vi "write RT config file.vi"(9 "RT config":T18={"Message"={"Parameters"={"FPGA Ref"=refnum, "configID"=0, "activeChannels"=[]}, "Variables"={"RT Status"={"Comms loop"=FALSE, "scheduler loop"=FALSE, "data process loop"=FALSE, "FIFO loop"=FALSE, "Command Stream"=FALSE, "Error Stream"=FALSE, "FPGA FIFO"=FALSE, "Data Stream"=FALSE}, "watchdog"=timestamp(0 s since 1904-01-01), "limitsEnabled"=FALSE, "Interlocks"={"gearboxOil"=FALSE, "bearingOil"=FALSE, "gearboxAir"=FALSE}}}, "FIFO"={"Params"={"FPGA ref"=refnum, "Total Channels"=0}, "Variables"={"FIFO wait counter"=0, "FIFO read trigger"=0}}, "Comms data"={"Parameters"={"error writer name"="", "command reader name"="", "error buffer size"=0, "command buffer size"=0, "scanivalveIP"="", "scanivalvePeriod"=0}, "Variables"={"listen schedule"=0, "incident buffer"=[], "command stream"="", "error stream"="", "waiting for command stream connect"=FALSE, "waiting for error stream connect"=FALSE, "scanivalve connection"=refnum, "scanivalveScheduleID"=0, "activeScanivalvePorts"=[], "channelCount"=0}, "scanivalveConfig"={"listS"={"period"=0, "ADtrig"=FALSE, "ScanTrig"=FALSE, "page"=0, "qpkts"=0}, "listC"={"ZC"=FALSE, "unitScan"="", "CvtUnit"=0.0, "bin"=FALSE, "EU"=FALSE}, "listSG"={"Avg1"=0, "FPS1"=0, "SGEnable1"=FALSE}, "activeChannels"={"Chan1"={"101"=FALSE, "102"=FALSE, "103"=FALSE, "104"=FALSE, "109"=FALSE, "110"=FALSE, "111"=FALSE, "112"=FALSE, "201"=FALSE, "202"=FALSE, "203"=FALSE, "204"=FALSE, "209"=FALSE, "210"=FALSE, "211"=FALSE, "212"=FALSE, "301"=FALSE, "302"=FALSE, "303"=FALSE, "304"=FALSE, "309"=FALSE, "310"=FALSE, "311"=FALSE, "312"=FALSE, "401"=FALSE, "402"=FALSE, "403"=FALSE, "404"=FALSE, "409"=FALSE, "410"=FALSE, "411"=FALSE, "412"=FALSE}}}}, "Data processor"={"Parameters"={"FPGA Ref"=refnum, "data stream"={"data writer name"="error writer", "NS write buffer size"=16, "NS Buffer length"=0}, "FIFO Depth"=0, "Channel controls"={"FIFO channel count"=0, "active indices"=[], "active channels"=0, "channelScaling"=[], "scanivalveCount"=0, "channels"=[]}, "safetyChannels"={"oilP"=0, "airP"=0, "water"=0, "channelLimits"=[]}, "speedChannel"=0, "maxSpeedLimit"=0.0, "Torque"={"fixedOffset"=0.0, "filter"=FALSE, "fallingEdge"=FALSE, "swapEncoders"=FALSE}}, "Variables"={"Intermediary buffer"=[], "buffer position"=0, "write loop counter"=0, "NS write trigger"=0, "NS Connection status"=FALSE, "waiting for NS"=FALSE, "labAmbient"={"pressure"=0.0, "temperature"=0.0}, "scanivalvePorts"=[], "scanivalvePressures"=[], "data stream"="", "activeChannelLimitIndex"=[], "runningSpeedLimit"=0.0, "speedChannelIndex"=0, "Interlocks"={"gearboxOil"=FALSE, "bearingOil"=FALSE, "gearboxAir"=FALSE}, "interlockChannels"={"gearboxOil"=0, "bearingOil"=0, "air"=0}, "limitStates"=[]}}}, 11 "RT config file path":path) -> ()   [LabVIEW 2018]
uses:
  RT/Type Defs/Message loop data.ctl
  RT/Type Defs/FPGA reference.ctl
  RT/Type Defs/RT Status.ctl
  RT/Type Defs/Analogue loop data.ctl
  RT/Communications loop/comms data.ctl
  RT/Type Defs/generic incident.ctl
  ICL-LabVIEW_General/Scanivalve API project/full interface/polymorphic/scanivalveConfig.ctl
  ICL-LabVIEW_General/Scanivalve API project/full interface/listS.ctl
  ICL-LabVIEW_General/Scanivalve API project/full interface/listC.ctl
  ICL-LabVIEW_General/Scanivalve API project/full interface/listSG.ctl
  ICL-LabVIEW_General/Scanivalve API project/full interface/chan1.ctl
  RT/Type Defs/Data processing loop data.ctl
  type defs/channelControl.ctl
  RT/Type Defs/channelScalingTypes.ctl
  RT/Type Defs/scalingMethods.ctl
  ICL-LabVIEW_General/data channels/parent class/Data Channel.lvclass
  type defs/channelLimitControl.ctl
  type defs/limitActions.ctl
  <vilib>/Utility/config.llb/Write Key (U32).vi
  <vilib>/Utility/config.llb/Write Key (I32).vi
  <vilib>/Utility/config.llb/Write Key (String).vi
  <vilib>/Utility/config.llb/Write Key (Double).vi
  <vilib>/Utility/config.llb/Write Key (Boolean).vi
  <vilib>/Utility/config.llb/NI_LVConfig.lvlib
  ICL-LabVIEW_General/Scanivalve API project/Scanivalve API.lvlib
panel:
  out "unwritten keys":string[](array[string])
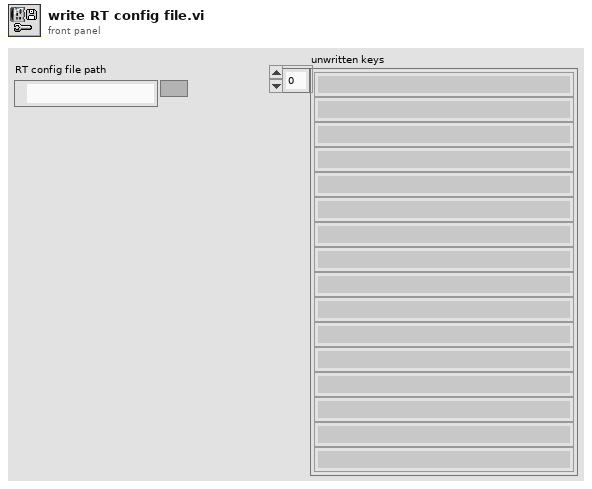
[diagram p1: front panel]
types:
  T1 = typedef "Message loop data.ctl" = cluster{"Parameters":cluster{"FPGA Ref":T2, "configID":u32, "activeChannels":cluster{"index":u16, "name":string}[]}, "Variables":cluster{"RT Status":T3, "watchdog":timestamp, "limitsEnabled":bool, "Interlocks":cluster{"gearboxOil":bool, "bearingOil":bool, "gearboxAir":bool}}}
  T2 = typedef "FPGA reference.ctl" = refnum<k20>
  T3 = typedef "RT Status.ctl" = cluster{"Comms loop":bool, "scheduler loop":bool, "data process loop":bool, "FIFO loop":bool, "Command Stream":bool, "Error Stream":bool, "FPGA FIFO":bool, "Data Stream":bool}
  T4 = typedef "Analogue loop data.ctl" = cluster{"Params":cluster{"FPGA ref":T2, "Total Channels":u32}, "Variables":cluster{"FIFO wait counter":u16, "FIFO read trigger":u32}}
  T5 = typedef "comms data.ctl" = cluster{"Parameters":cluster{"error writer name":string, "command reader name":string, "error buffer size":i32, "command buffer size":i32, "scanivalveIP":string, "scanivalvePeriod":u16}, "Variables":cluster{"listen schedule":u32, "incident buffer":T6[], "command stream":refnum<k21>, "error stream":refnum<k21>, "waiting for command stream connect":bool, "waiting for error stream connect":bool, "scanivalve connection":refnum<k5>, "scanivalveScheduleID":u32, "activeScanivalvePorts":i32[], "channelCount":i16}, "scanivalveConfig":T7}
  T6 = typedef "generic incident.ctl" = cluster{"timestamp":timestamp, "type":string, "Variant":variant}
  T7 = typedef "Scanivalve API.lvlib/scanivalveConfig.ctl" = cluster{"listS":T8, "listC":T9, "listSG":T10, "activeChannels":T11}
  T8 = typedef "Scanivalve API.lvlib/listS.ctl" = cluster{"period":u16, "ADtrig":bool, "ScanTrig":bool, "page":u16, "qpkts":u16}
  T9 = typedef "Scanivalve API.lvlib/listC.ctl" = cluster{"ZC":bool, "unitScan":string, "CvtUnit":dbl, "bin":bool, "EU":bool}
  T10 = typedef "Scanivalve API.lvlib/listSG.ctl" = cluster{"Avg1":u16, "FPS1":u16, "SGEnable1":bool}
  T11 = typedef "Scanivalve API.lvlib/chan1.ctl" = cluster{"Chan1":cluster{"101":bool, "102":bool, "103":bool, "104":bool, "109":bool, "110":bool, "111":bool, "112":bool, "201":bool, "202":bool, "203":bool, "204":bool, "209":bool, "210":bool, "211":bool, "212":bool, "301":bool, "302":bool, "303":bool, "304":bool, "309":bool, "310":bool, "311":bool, "312":bool, "401":bool, "402":bool, "403":bool, "404":bool, "409":bool, "410":bool, "411":bool, "412":bool}}
  T12 = typedef "Data processing loop data.ctl" = cluster{"Parameters":cluster{"FPGA Ref":T2, "data stream":cluster{"data writer name":string, "NS write buffer size":i32, "NS Buffer length":u32}, "FIFO Depth":u32, "Channel controls":cluster{"FIFO channel count":i32, "active indices":i16[], "active channels":i32, "channelScaling":T13[], "scanivalveCount":i32, "channels":refnum<class "Data Channel.lvclass">[]}, "safetyChannels":cluster{"oilP":u16, "airP":u16, "water":u16, "channelLimits":T16[]}, "speedChannel":i32, "maxSpeedLimit":dbl, "Torque":cluster{"fixedOffset":dbl, "filter":bool, "fallingEdge":bool, "swapEncoders":bool}}, "Variables":cluster{"Intermediary buffer":dbl[][], "buffer position":u32, "write loop counter":u16, "NS write trigger":u32, "NS Connection status":bool, "waiting for NS":bool, "labAmbient":cluster{"pressure":dbl, "temperature":dbl}, "scanivalvePorts":u16[], "scanivalvePressures":dbl[], "data stream":refnum<k21>, "activeChannelLimitIndex":u16[], "runningSpeedLimit":dbl, "speedChannelIndex":i32, "Interlocks":cluster{"gearboxOil":bool, "bearingOil":bool, "gearboxAir":bool}, "interlockChannels":cluster{"gearboxOil":i32, "bearingOil":i32, "air":i32}, "limitStates":cluster{"warn":bool, "alarm":bool}[]}}
  T13 = typedef "channelControl.ctl" = cluster{"index":u16, "active":bool, "channelType":T14, "module":u16, "terminal":u16, "channelName":string, "scalingMethod":T15, "scalingParameters":dbl[], "scaledUnits":string, "tempOffset":dbl}
  T14 = typedef "channelScalingTypes.ctl" = enum16{"calculation", "measurement", "scanivalve", "output", "digital"}
  T15 = typedef "scalingMethods.ctl" = enum16{"none", "linear", "thermocouple", "polynomial", "encoder", "RTD"}
  T16 = typedef "channelLimitControl.ctl" = cluster{"channelID":u16, "Enabled":bool, "warnValue":dbl, "limitValue":dbl, "Invert":bool, "limitAction":T17}
  T17 = typedef "limitActions.ctl" = enum16{"stop", "shutdown", "ignore"}
  T18 = cluster{"Message":T1, "FIFO":T4, "Comms data":T5, "Data processor":T12}
  T19 = typedef "NI_LVConfig.lvlib/Config Data RefNum.ctl" = refnum<k1>
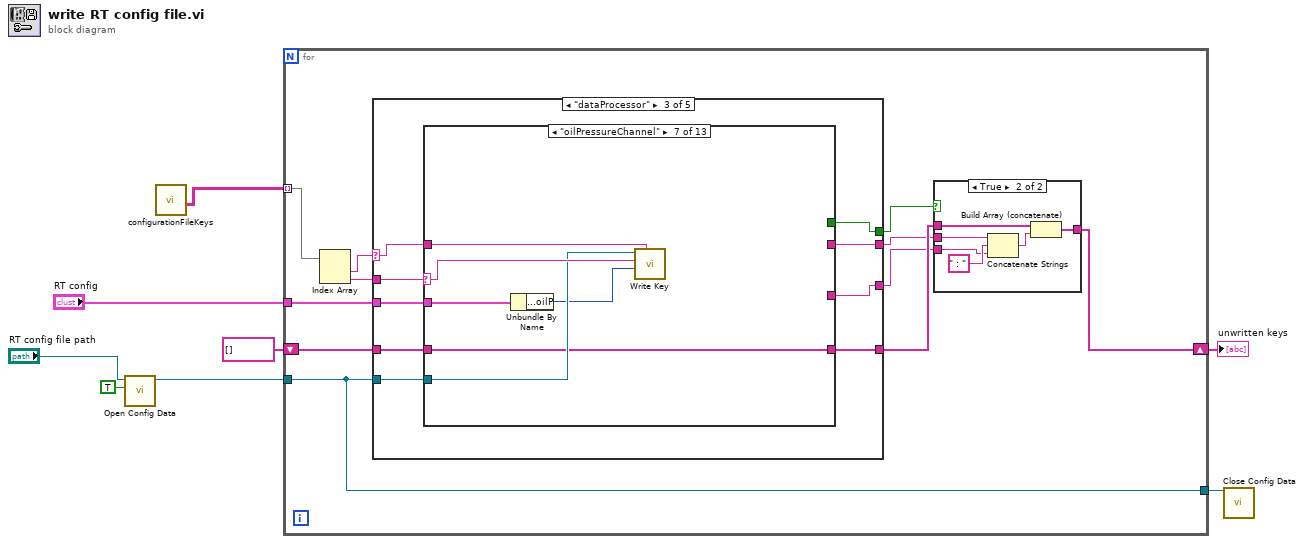
[diagram p0: block diagram]
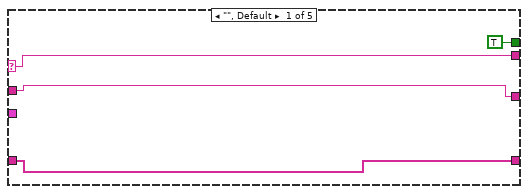
[diagram p3: hidden frame]
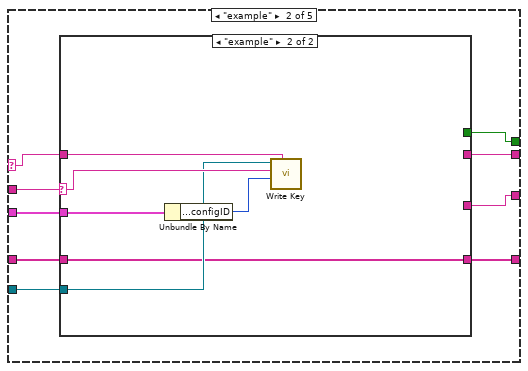
[diagram p4: hidden frame]
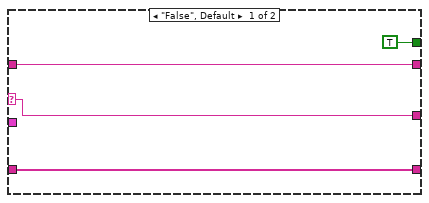
[diagram p5: hidden frame]
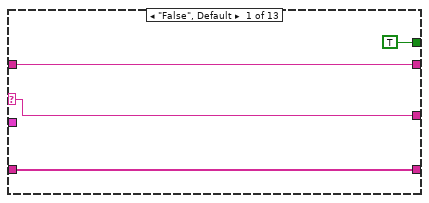
[diagram p6: hidden frame]
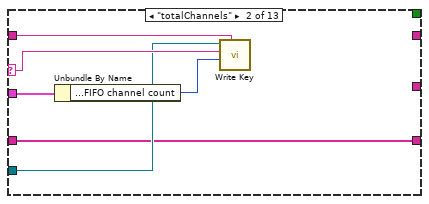
[diagram p7: hidden frame]
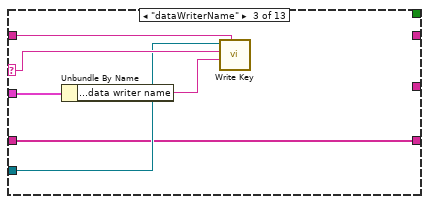
[diagram p8: hidden frame]
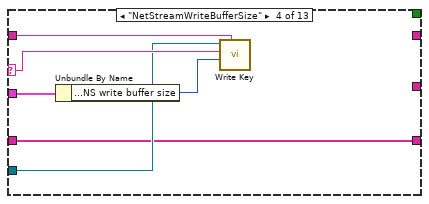
[diagram p9: hidden frame]
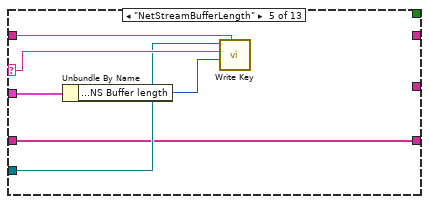
[diagram p10: hidden frame]
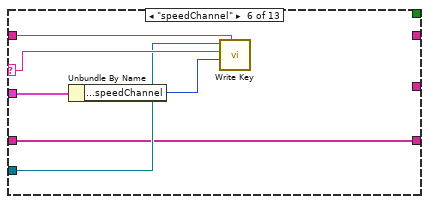
[diagram p11: hidden frame]
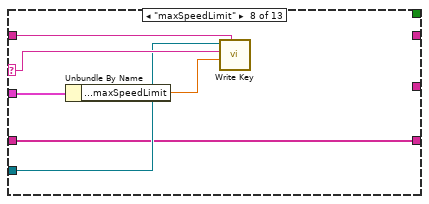
[diagram p12: hidden frame]
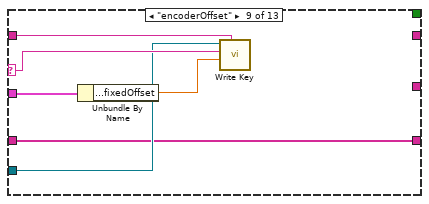
[diagram p13: hidden frame]
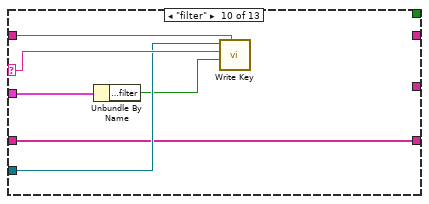
[diagram p14: hidden frame]
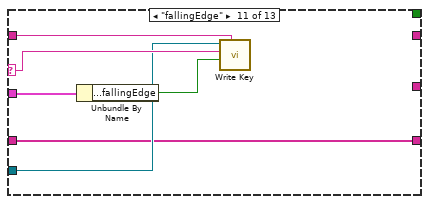
[diagram p15: hidden frame]
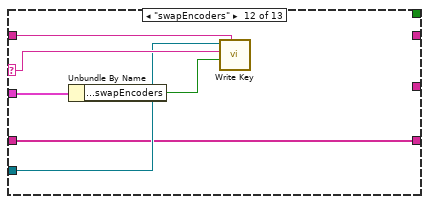
[diagram p16: hidden frame]
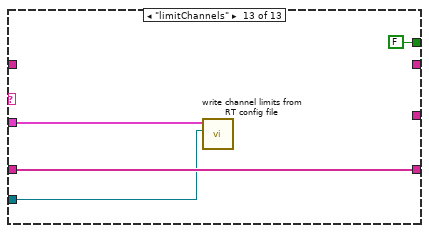
[diagram p17: hidden frame]
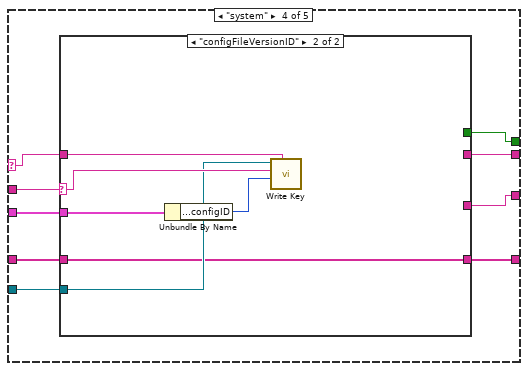
[diagram p18: hidden frame]
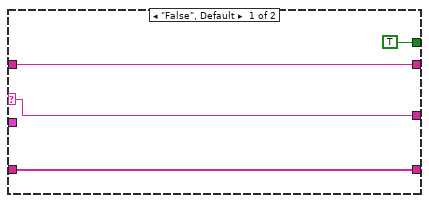
[diagram p19: hidden frame]
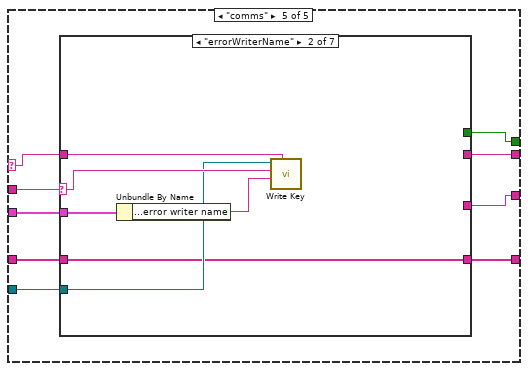
[diagram p20: hidden frame]
diagram:
  n1 = call <vilib>:"Open Config Data.vi"("create file if necessary (T)"=TRUE, "configuration file path"="RT config file path") -> ("refnum"=w8:T19)  [unwired: 7 in, 2 out]
  n2 = call "configurationFileKeys.vi"() -> ("configKeysRT"=w2:string[][])  [unwired: 9 in, 2 out]
  n3 = for {
    tunnel: "RT config" -> [w15]
    tunnel: w2 -> [w19] mode=indexing
    tunnel: w8 -> [w16]
    tunnel: [w16] -> w7
    shift-right: [w12] -> w4
    shift-left: string[] [] -> [w14]
    n4 = Index Array(array=w19) -> (element #1=w18:string, element #2=w17:string)  [unwired: 2 in]
    n5 = case shown="\"dataProcessor\"" w18 {
      selector: w18 -> [w30 w36 w55 w138 w157]
      tunnel: w17 -> [w29 w39 w58 w141 w160]
      tunnel: w16 -> [_ w38 w57 w140 w159]
      tunnel: w15 -> [_ w37 w56 w139 w158]
      tunnel: [w28 w35 w54 w137 w156] -> w13
      tunnel: w14 -> [w28 w34 w53 w136 w155]
      tunnel: [TRUE w31 w50 w133 w152] -> w9
      tunnel: [w30 w33 w52 w135 w154] -> w11
      tunnel: [w29 w32 w51 w134 w153] -> w10
      frame "", Default {
      }
      frame "example" {
        n6 = case shown="\"example\"" w39 {
          selector: w39 -> [w41 w48]
          tunnel: w38 -> [_ w47]
          tunnel: w37 -> [_ w46]
          tunnel: w36 -> [w42 w49]
          tunnel: [w43 w44] -> w35
          tunnel: w34 -> [w43 w44]
          tunnel: [w42 _] -> w33
          tunnel: [w41 _] -> w32
          tunnel: [TRUE _] -> w31
          frame "False", Default {
          }
          frame "example" {
            n7 = Unbundle By Name(w46) -> ("Message.Parameters.configID"=w45:u32)
            n8 = call-poly <vilib>:"Write Key.vi"("section"=w49, "value"=w45, "key"=w48, "refnum"=w47) -> ()  [unwired: 5 in, 3 out]
          }
        }
      }
      frame "dataProcessor" {
        n9 = case shown="\"oilPressureChannel\"" w58 {
          selector: w58 -> [w60 w67 w73 w79 w85 w91 w97 w103 w109 w115 w121 w127 _]
          tunnel: w57 -> [_ w66 w72 w78 w84 w90 w96 w102 w108 w114 w120 w126 w129]
          tunnel: w56 -> [_ w65 w71 w77 w83 w89 w95 w101 w107 w113 w119 w125 w132]
          tunnel: w55 -> [w61 w68 w74 w80 w86 w92 w98 w104 w110 w116 w122 w128 _]
          tunnel: [w62 w63 w69 w75 w81 w87 w93 w99 w105 w111 w117 w123 w130] -> w54
          tunnel: w53 -> [w62 w63 w69 w75 w81 w87 w93 w99 w105 w111 w117 w123 w130]
          tunnel: [w61 _ _ _ _ _ _ _ _ _ _ _ _] -> w52
          tunnel: [w60 _ _ _ _ _ _ _ _ _ _ _ _] -> w51
          tunnel: [TRUE _ _ _ _ _ _ _ _ _ _ _ FALSE] -> w50
          frame "False", Default {
          }
          frame "totalChannels" {
            n10 = Unbundle By Name(w65) -> ("Data processor.Parameters.Channel controls.FIFO channel count"=w64:i32)
            n11 = call-poly <vilib>:"Write Key.vi"("section"=w68, "value"=w64, "key"=w67, "refnum"=w66) -> ()  [unwired: 5 in, 3 out]
          }
          frame "dataWriterName" {
            n12 = Unbundle By Name(w71) -> ("Data processor.Parameters.data stream.data writer name"=w70:string)
            n13 = call-poly <vilib>:"Write Key.vi"("section"=w74, "value"=w70, "key"=w73, "refnum"=w72) -> ()  [unwired: 5 in, 3 out]
          }
          frame "NetStreamWriteBufferSize" {
            n14 = Unbundle By Name(w77) -> ("Data processor.Parameters.data stream.NS write buffer size"=w76:i32)
            n15 = call-poly <vilib>:"Write Key.vi"("section"=w80, "value"=w76, "key"=w79, "refnum"=w78) -> ()  [unwired: 5 in, 3 out]
          }
          frame "NetStreamBufferLength" {
            n16 = Unbundle By Name(w83) -> ("Data processor.Parameters.data stream.NS Buffer length"=w82:u32)
            n17 = call-poly <vilib>:"Write Key.vi"("section"=w86, "value"=w82, "key"=w85, "refnum"=w84) -> ()  [unwired: 5 in, 3 out]
          }
          frame "speedChannel" {
            n18 = Unbundle By Name(w89) -> ("Data processor.Parameters.speedChannel"=w88:i32)
            n19 = call-poly <vilib>:"Write Key.vi"("section"=w92, "value"=w88, "key"=w91, "refnum"=w90) -> ()  [unwired: 5 in, 3 out]
          }
          frame "oilPressureChannel" {
            n20 = Unbundle By Name(w95) -> ("Data processor.Parameters.safetyChannels.oilP"=w94:u16)
            n21 = call-poly <vilib>:"Write Key.vi"("section"=w98, "value"=w94, "key"=w97, "refnum"=w96) -> ()  [unwired: 5 in, 3 out]
          }
          frame "maxSpeedLimit" {
            n22 = Unbundle By Name(w101) -> ("Data processor.Parameters.maxSpeedLimit"=w100:dbl)
            n23 = call-poly <vilib>:"Write Key.vi"("section"=w104, "value"=w100, "key"=w103, "refnum"=w102) -> ()  [unwired: 5 in, 3 out]
          }
          frame "encoderOffset" {
            n24 = Unbundle By Name(w107) -> ("Data processor.Parameters.Torque.fixedOffset"=w106:dbl)
            n25 = call-poly <vilib>:"Write Key.vi"("section"=w110, "value"=w106, "key"=w109, "refnum"=w108) -> ()  [unwired: 5 in, 3 out]
          }
          frame "filter" {
            n26 = Unbundle By Name(w113) -> ("Data processor.Parameters.Torque.filter"=w112:bool)
            n27 = call-poly <vilib>:"Write Key.vi"("section"=w116, "value"=w112, "key"=w115, "refnum"=w114) -> ()  [unwired: 5 in, 3 out]
          }
          frame "fallingEdge" {
            n28 = Unbundle By Name(w119) -> ("Data processor.Parameters.Torque.fallingEdge"=w118:bool)
            n29 = call-poly <vilib>:"Write Key.vi"("section"=w122, "value"=w118, "key"=w121, "refnum"=w120) -> ()  [unwired: 5 in, 3 out]
          }
          frame "swapEncoders" {
            n30 = Unbundle By Name(w125) -> ("Data processor.Parameters.Torque.swapEncoders"=w124:bool)
            n31 = call-poly <vilib>:"Write Key.vi"("section"=w128, "value"=w124, "key"=w127, "refnum"=w126) -> ()  [unwired: 5 in, 3 out]
          }
          frame "limitChannels" {
            n32 = call "write channel limits from RT config file.vi"("configFileRef"=w129, "RT config"=w132) -> ()  [unwired: 10 in]
          }
        }
      }
      frame "system" {
        n33 = case shown="\"configFileVersionID\"" w141 {
          selector: w141 -> [w143 w150]
          tunnel: w140 -> [_ w149]
          tunnel: w139 -> [_ w148]
          tunnel: w138 -> [w144 w151]
          tunnel: [w145 w146] -> w137
          tunnel: w136 -> [w145 w146]
          tunnel: [w144 _] -> w135
          tunnel: [w143 _] -> w134
          tunnel: [TRUE _] -> w133
          frame "False", Default {
          }
          frame "configFileVersionID" {
            n34 = Unbundle By Name(w148) -> ("Message.Parameters.configID"=w147:u32)
            n35 = call-poly <vilib>:"Write Key.vi"("section"=w151, "value"=w147, "key"=w150, "refnum"=w149) -> ()  [unwired: 5 in, 3 out]
          }
        }
      }
      frame "comms" {
        n36 = case shown="\"errorWriterName\"" w160 {
          selector: w160 -> [w162 w169 w175 w181 w187 w193 w199]
          tunnel: w159 -> [_ w168 w174 w180 w186 w192 w198]
          tunnel: w158 -> [_ w167 w173 w179 w185 w191 w197]
          tunnel: w157 -> [w163 w170 w176 w182 w188 w194 w200]
          tunnel: [w164 w165 w171 w177 w183 w189 w195] -> w156
          tunnel: w155 -> [w164 w165 w171 w177 w183 w189 w195]
          tunnel: [w163 _ _ _ _ _ _] -> w154
          tunnel: [w162 _ _ _ _ _ _] -> w153
          tunnel: [TRUE _ _ _ _ _ _] -> w152
          frame "False", Default {
          }
          frame "errorWriterName" {
            n37 = Unbundle By Name(w167) -> ("Comms data.Parameters.error writer name"=w166:string)
            n38 = call-poly <vilib>:"Write Key.vi"("section"=w170, "value"=w166, "key"=w169, "refnum"=w168) -> ()  [unwired: 5 in, 3 out]
          }
          frame "commandReaderName" {
            n39 = Unbundle By Name(w173) -> ("Comms data.Parameters.command reader name"=w172:string)
            n40 = call-poly <vilib>:"Write Key.vi"("section"=w176, "value"=w172, "key"=w175, "refnum"=w174) -> ()  [unwired: 5 in, 3 out]
          }
          frame "errorBufferSize" {
            n41 = Unbundle By Name(w179) -> ("Comms data.Parameters.error buffer size"=w178:i32)
            n42 = call-poly <vilib>:"Write Key.vi"("section"=w182, "value"=w178, "key"=w181, "refnum"=w180) -> ()  [unwired: 5 in, 3 out]
          }
          frame "commandBufferSize" {
            n43 = Unbundle By Name(w185) -> ("Comms data.Parameters.command buffer size"=w184:i32)
            n44 = call-poly <vilib>:"Write Key.vi"("section"=w188, "value"=w184, "key"=w187, "refnum"=w186) -> ()  [unwired: 5 in, 3 out]
          }
          frame "scanivalveIP" {
            n45 = Unbundle By Name(w191) -> ("Comms data.Parameters.scanivalveIP"=w190:string)
            n46 = call-poly <vilib>:"Write Key.vi"("section"=w194, "value"=w190, "key"=w193, "refnum"=w192) -> ()  [unwired: 5 in, 3 out]
          }
          frame "scanPeriod" {
            n47 = Unbundle By Name(w197) -> ("Comms data.Parameters.scanivalvePeriod"=w196:u16)
            n48 = call-poly <vilib>:"Write Key.vi"("section"=w200, "value"=w196, "key"=w199, "refnum"=w198) -> ()  [unwired: 5 in, 3 out]
          }
        }
      }
    }
    n49 = case shown="True" w9 {
      tunnel: [w20 w23] -> w12
      tunnel: w13 -> [w20 w24]
      tunnel: w11 -> [_ w22]
      tunnel: w10 -> [_ w21]
      frame False {
      }
      frame True {
        n50 = Concatenate Strings(w22, " : " ("string"), w21) -> (w25:string)
        n51 = Build Array (concatenate)(w24, w25) -> (w23:string[])
      }
    }
  }
  "unwritten keys" <- w4
  n52 = call <vilib>:"Close Config Data.vi"("refnum"=w7) -> ()  [unwired: 9 in, 2 out]
